vi "set channel settings id.vi"(8 "error in (no error)":errorcluster, 9 "settings id":string, 10 "id":string, 11 "DSFConfiguration in":refnum<class "DSFConfiguration.lvclass">) -> (0 "error out":errorcluster, 3 "DSFConfiguration out":refnum<class "DSFConfiguration.lvclass">)   [LabVIEW 2017, in "DSFConfiguration.lvclass"]
uses:
  DSFConfiguration.lvclass
  IDable/IDable.lvclass
  DSFChannel/DSFChannel.lvclass
  C:/github/data-sharing-framework-custom-device/Source/Submodules/DSF/Source/Configuration API/Classes/IDable/IDable.lvclass
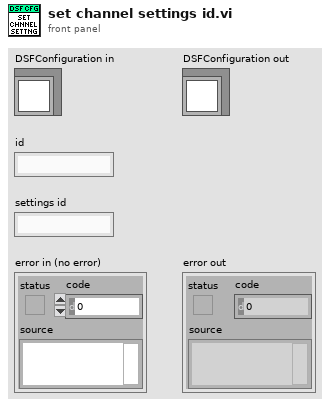
[diagram p1: front panel]
types:
  T1 = typedef "dsf configuration file v1.0.0.lvlib/dsf channel.ctl" = cluster{"id":string, "values":cluster{"count":i32, "offset":i32, "data type":dbl, "resource path":string, "settings":string}}
  T2 = typedef "dsf configuration file v1.0.0.lvlib/dsf settings.ctl" = cluster{"id":string, "values":cluster{"key":string, "value":string}[]}
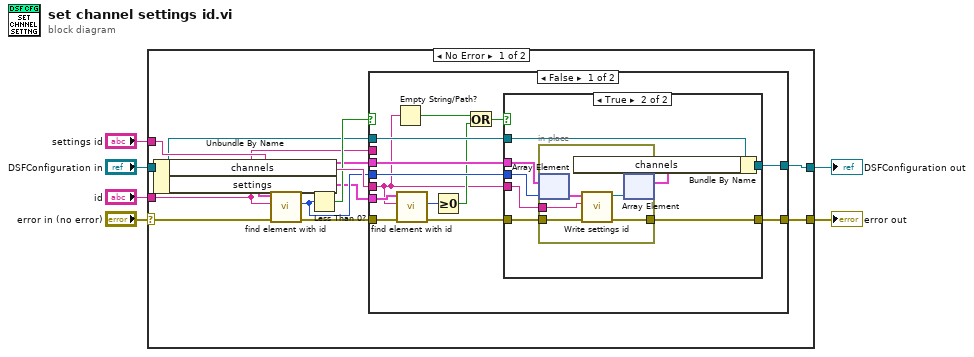
[diagram p0: block diagram]
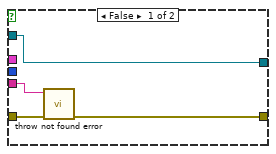
[diagram p2: hidden frame]
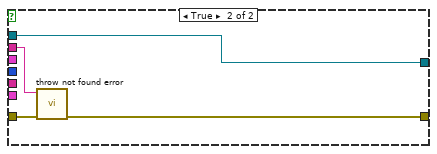
[diagram p3: hidden frame]
diagram:
  n1 = case shown="No Error" "error in (no error)" {
    selector: "error in (no error)" -> [w17 w53]
    tunnel: [w16 w53] -> w5
    tunnel: [w8 w52] -> w3
    tunnel: "DSFConfiguration in" -> [w9 w52]
    tunnel: "id" -> [w7 _]
    tunnel: "settings id" -> [w15 _]
    frame No Error {
      n2 = Unbundle By Name(w9) -> ("channels"=w12:T1[], "settings"=w10:T2[])
      n3 = call "find element with id.vi"("error in (no error)"=w17, "id"=w7, "IDable Array in"=w12) -> ("error out"=w13:errorcluster, "index"=w11:i32)  [unwired: 7 in]
      n4 = Less Than 0?(x=w11) -> (x < 0?=w14:bool)
      n5 = case shown="False" w14 {
        tunnel: w13 -> [w23 w48]
        tunnel: [w28 w51] -> w16
        tunnel: w12 -> [w30 _]
        tunnel: w11 -> [w29 _]
        tunnel: w15 -> [w20 _]
        tunnel: [w27 w50] -> w8
        tunnel: w10 -> [w26 _]
        tunnel: w9 -> [w24 w50]
        tunnel: w7 -> [_ w49]
        frame False {
          n6 = Empty String/Path?(string/path=w20) -> (empty?=w18:bool)
          n7 = call "find element with id.vi"("error in (no error)"=w23, "id"=w20, "IDable Array in"=w26) -> ("error out"=w22:errorcluster, "index"=w25:i32)  [unwired: 7 in]
          n8 = Greater Or Equal To 0?(x=w25) -> (x >= 0?=w21:bool)
          n9 = Or(x=w18, y=w21) -> (x .or. y?=w19:bool)
          n10 = case shown="True" w19 {
            tunnel: w30 -> [_ w42]
            tunnel: w29 -> [_ w41]
            tunnel: w22 -> [w31 w40]
            tunnel: [w33 w39] -> w28
            tunnel: [w34 w36] -> w27
            tunnel: w20 -> [w32 w38]
            tunnel: w24 -> [w34 w37]
            frame False {
              n11 = call "throw not found error.vi"("error in (no error)"=w31, "id"=w32) -> ("error out"=w33:errorcluster)  [unwired: 9 in]
            }
            frame True {
              n12 = in-place {
                in-place-border: w38 -> [w43]
                in-place-border: w40 -> [w47]
                in-place-border: [w46] -> w39
                n13 = in-place-array #1(w42, w41) -> (w45:T1)
                n14 = call "Write settings id.vi"("error in (no error)"=w47, "settings id"=w43, "DSFChannel in"=w45) -> ("error out"=w46:errorcluster, "DSFChannel out"=w44:refnum<class "DSFChannel.lvclass">)  [unwired: 7 in]
                n15 = in-place-array #1(w44) -> (w35:T1[])  [unwired: 1 out]
              }
              n16 = Bundle By Name(cluster=w37, "channels"=w35) -> (w36:refnum<class "DSFConfiguration.lvclass">)
            }
          }
        }
        frame True {
          n17 = call "throw not found error.vi"("error in (no error)"=w48, "id"=w49) -> ("error out"=w51:errorcluster)  [unwired: 9 in]
        }
      }
    }
    frame Error {
    }
  }
  "error out" <- w5
  "DSFConfiguration out" <- w3
